vi "C-R Speed Test AIN eNames LJMIntervals.vi"() -> ()   [LabVIEW 2020]
panel:
  in  "Interval [ms]":ext format="%.3f"
  out "Interval Array (Sorted Descending)":ext[](array[numeric]) format="%.3g"
  in  "Range":dbl=10.0 format="%.2f"
  out "ConnectionType Out":i32
  out "DeviceType Out":i32
  in  "Identifier":string="LJM_idANY"
  in  "ConnectionType":string="LJM_ctANY"
  in  "DeviceType":string="LJM_dtANY"
  in  "Enable Interval Timing":bool
  out "min ms":ext format="%.3g"
  out "max ms":ext format="%.3g"
  out "avg ms per iteration":ext format="%.3f"
  out "Interval Array":ext[](array[numeric]) format="%.3g"
  in  "Write Both DACs":bool
  in  "Write Digital":bool
  in  "Read Digital":bool
  out "total ms":ext format="%.3g"
  in  "# Iterations":i32=1000
  in  "# AIN Channels":i32=1
  in  "Settling":i32
  out "Error Message":string
  in  "Resolution Index":i32=1
  out "error out":errorcluster
  # "This variation of the speed test VI uses our GetHostTick function with\nmicrosecond resolution, rather than LabVIEW's Tick Count funtion with\nmillisecond resolution."
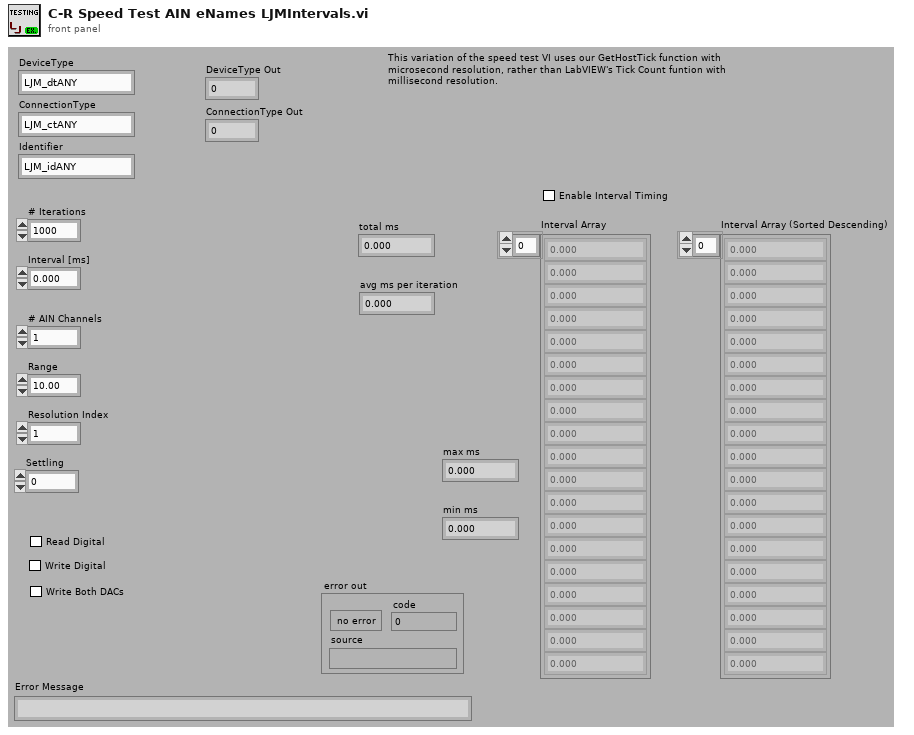
[diagram p1: front panel]
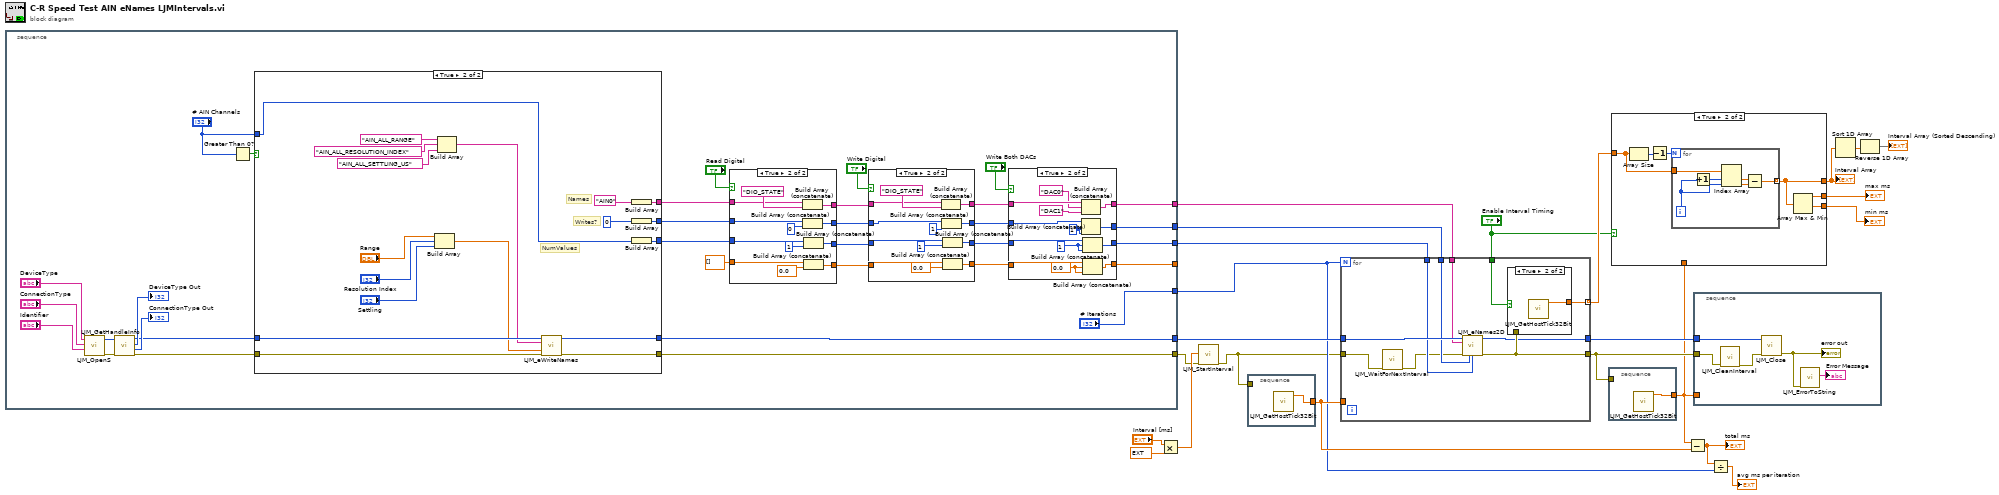
[diagram p0: block diagram]
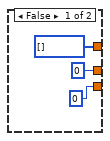
[diagram p2: hidden frame]
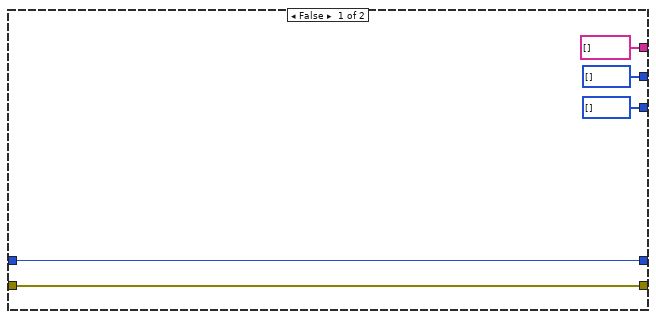
[diagram p3: hidden frame]
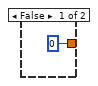
[diagram p7: hidden frame]
diagram:
  n1 = stacked-sequence {
    tunnel: [w35] -> w23
    tunnel: [w25] -> w2
    tunnel: ["# Iterations"] -> w18
    tunnel: [w28] -> w15
    tunnel: [w27] -> w14
    tunnel: [w26] -> _
    tunnel: [w24] -> w9
    frame #0 {
      n2 = call "LJM_OpenS.vi"("Identifier"="Identifier", "ConnectionType"="ConnectionType", "DeviceType"="DeviceType") -> ("error out"=w42:errorcluster, "Handle"=w43:i32)  [unwired: 7 in]
      n3 = call "LJM_GetHandleInfo.vi"("error in"=w42, "Handle In"=w43) -> ("error out"=w36:errorcluster, "ConnectionType"=→"ConnectionType Out":i32, "DeviceType"=→"DeviceType Out":i32, "Handle Out"=w37:i32)  [unwired: 2 in, 4 out]
      n4 = Greater Than 0?(x="# AIN Channels") -> (x > 0?=w39:bool)
      n5 = case shown="True" w39 {
        tunnel: "# AIN Channels" -> [_ w69]
        tunnel: w37 -> [w61 w79]
        tunnel: w36 -> [w60 w78]
        tunnel: [w60 w77] -> w25
        tunnel: [w61 w76] -> w35
        tunnel: [string[] [] w71] -> w34
        tunnel: [i32[] [] w70] -> w33
        tunnel: [i32[] [] w68] -> w31
        frame False {
        }
        frame True {
          # "NumValues"
          # "Names"
          # "Writes?"
          n6 = Build Array("Range", "Resolution Index", "Settling") -> (w75:dbl[])
          n7 = Build Array("AIN_ALL_RANGE" ("Substring"), "AIN_ALL_RESOLUTION_INDEX" ("Substring"), "AIN_ALL_SETTLING_US" ("Substring")) -> (w74:string[])
          n8 = call "LJM_eWriteNames.vi"("Handle In"=w79, "aNames"=w74, "aValuesIn"=w75, "error in"=w78) -> ("Handle Out"=w76:i32, "error out"=w77:errorcluster)  [unwired: 9 in, 1 out]
          n9 = Build Array("AIN0") -> (w71:string[])
          n10 = Build Array(0) -> (w70:i32[])
          n11 = Build Array(w69) -> (w68:i32[])
        }
      }
      n12 = case shown="True" "Read Digital" {
        tunnel: [w116 w123] -> w54
        tunnel: [w114 w125] -> w53
        tunnel: [w113 w124] -> w52
        tunnel: w34 -> [w116 w122]
        tunnel: w33 -> [w115 w121]
        tunnel: dbl[] [] ("Input Array") -> [w113 w120]
        tunnel: w31 -> [w114 w119]
        tunnel: [w115 w118] -> w30
        frame False {
        }
        frame True {
          n13 = Build Array (concatenate)(w122, "DIO_STATE" ("IOType")) -> (w123:string[])
          n14 = Build Array (concatenate)(w121, 0) -> (w118:i32[])
          n15 = Build Array (concatenate)(w119, 1) -> (w125:i32[])
          n16 = Build Array (concatenate)(w120, 0.0) -> (w124:dbl[])
        }
      }
      n17 = case shown="True" "Write Digital" {
        tunnel: [w100 w112] -> w51
        tunnel: w54 -> [w100 w110]
        tunnel: [w99 w106] -> w50
        tunnel: w53 -> [w99 w109]
        tunnel: w52 -> [w98 w105]
        tunnel: [w98 w104] -> w49
        tunnel: w30 -> [w97 w103]
        tunnel: [w97 w101] -> w29
        frame False {
        }
        frame True {
          n18 = Build Array (concatenate)(w110, "DIO_STATE" ("IOType")) -> (w112:string[])
          n19 = Build Array (concatenate)(w103, 1) -> (w101:i32[])
          n20 = Build Array (concatenate)(w109, 1) -> (w106:i32[])
          n21 = Build Array (concatenate)(w105, 0.0) -> (w104:dbl[])
        }
      }
      n22 = case shown="True" "Write Both DACs" {
        tunnel: [w83 w96] -> w24
        tunnel: w51 -> [w83 w95]
        tunnel: [w82 w93] -> w27
        tunnel: w50 -> [w82 w94]
        tunnel: w49 -> [w81 w92]
        tunnel: [w81 w91] -> w26
        tunnel: w29 -> [w80 w85]
        tunnel: [w80 w84] -> w28
        frame False {
        }
        frame True {
          w86 = 1
          w89 = 0.0
          w90 = 1
          n23 = Build Array (concatenate)(w95, "DAC0" ("IOType"), "DAC1" ("Input Element")) -> (w96:string[])
          n24 = Build Array (concatenate)(w85, w86, w86) -> (w84:i32[])
          n25 = Build Array (concatenate)(w94, w90, w90) -> (w93:i32[])
          n26 = Build Array (concatenate)(w92, w89, w89) -> (w91:dbl[])
        }
      }
    }
  }
  n27 = Multiply(x="Interval [ms]", y=ext 1000.0) -> (x*y=w3:ext)
  n28 = call "LJM_StartInterval.vi"("error in"=w2, "Microseconds"=w3) -> ("error out"=w1:errorcluster)  [unwired: 9 in]
  n29 = stacked-sequence {
    tunnel: w1 -> [_]
    tunnel: [w129] -> w21
    frame #0 {
      n30 = call "LJM_GetHostTick32Bit.vi"() -> ("Tick Ext [ms]"=w129:ext)  [unwired: 9 in, 2 out]
    }
  }
  n31 = for {
    N: w18 -> [_]
    tunnel: w23 -> [w139]
    tunnel: w1 -> [w131]
    tunnel: [w137] -> w22
    tunnel: w21 -> [_]
    tunnel: "Enable Interval Timing" -> [w138]
    tunnel: [w136] -> w12 mode=indexing
    tunnel: w15 -> [w135]
    tunnel: w14 -> [w134]
    tunnel: [w133] -> w13
    tunnel: w9 -> [w132]
    n32 = call "LJM_WaitForNextInterval.vi"("error in"=w131) -> ("error out"=w130:errorcluster)  [unwired: 9 in, 1 out]
    n33 = call "LJM_eNames2D.vi"("Handle In"=w139, "aNames"=w132, "error in"=w130, "aWrites"=w135, "aNumValues"=w134) -> ("Handle Out"=w133:i32, "error out"=w137:errorcluster)  [unwired: 7 in, 2 out]
    n34 = case shown="True" w138 {
      tunnel: w137 -> [_ _]
      tunnel: [u32 0 ("millisecond timer value") w141] -> w136
      frame False {
      }
      frame True {
        n35 = call "LJM_GetHostTick32Bit.vi"() -> ("Tick Ext [ms]"=w141:ext)  [unwired: 9 in, 2 out]
      }
    }
  }
  n36 = stacked-sequence {
    tunnel: w22 -> [_]
    tunnel: [w142] -> w10
    frame #0 {
      n37 = call "LJM_GetHostTick32Bit.vi"() -> ("Tick Ext [ms]"=w142:ext)  [unwired: 9 in, 2 out]
    }
  }
  n38 = case shown="True" "Enable Interval Timing" {
    tunnel: [u32[] [] w149] -> w8
    tunnel: [u32 0 w148] -> w17
    tunnel: [u32 0 w147] -> w16
    tunnel: w12 -> [_ w146]
    tunnel: w10 -> [_ _]
    frame False {
    }
    frame True {
      n39 = Array Size(array=w146) -> (size(s)=w151:i32)
      n40 = Decrement(x=w151) -> (x-1=w150:i32)
      n41 = for {
        N: w150 -> [_]
        tunnel: w146 -> [w157]
        tunnel: [w152] -> w149 mode=indexing
        i -> [w155]
        n42 = Increment(x=w155) -> (x+1=w156:i32)
        n43 = Index Array(array=w157, index #1=w156, index #2=w155) -> (element #1=w153:ext, element #2=w154:ext)
        n44 = Subtract(x=w153, y=w154) -> (x-y=w152:ext)
      }
      n45 = Array Max & Min(array=w149) -> (max value=w148:ext, min value=w147:ext)  [unwired: 2 out]
    }
  }
  "Interval Array" <- w8
  "min ms" <- w16
  "max ms" <- w17
  n46 = Subtract(x=w10, y=w21) -> (x-y=w19:ext)
  "total ms" <- w19
  n47 = stacked-sequence {
    tunnel: w22 -> [w159]
    tunnel: w10 -> [_]
    tunnel: w13 -> [w160]
    frame #0 {
      n48 = call "LJM_CleanInterval.vi"("error in"=w159) -> ("error out"=w158:errorcluster)  [unwired: 10 in]
      n49 = call "LJM_Close.vi"("error in"=w158, "Handle"=w160) -> ("error out"=w161:errorcluster)  [unwired: 9 in]
      "error out" <- w161
      n50 = call "LJM_ErrorToString.vi"("error in"=w161) -> ("String"=→"Error Message":string)  [unwired: 10 in]
    }
  }
  n51 = Divide(x=w19, y=w18) -> (x/y=→"avg ms per iteration":ext)
  n52 = Sort 1D Array(array=w8) -> (sorted array=w7:ext[])
  n53 = Reverse 1D Array(array=w7) -> (reversed array=→"Interval Array (Sorted Descending)":ext[])
